vi "Find Songs By Artist.vi"(8 "error in (no error)":errorcluster, 10 "Artist":string, 11 "MusicLibrary in":refnum<class "MusicLibrary.lvclass">) -> (0 "error out":errorcluster, 2 "Songs":refnum<class "Song.lvclass">[](array[class]), 3 "MusicLibrary out":refnum<class "MusicLibrary.lvclass">, 5 "Found?":bool)   [LabVIEW 2015, in "MusicLibrary.lvclass"]
uses:
  MusicLibrary.lvclass
  Song/Song.lvclass
  MusicElementLibrary.lvclass/MusicElementLibrary.ctl
  SongLibrary/SongLibrary.lvclass
  Album/Album.lvclass/Album.ctl
  Song/Song.lvclass/Song.ctl
  MusicElement.lvclass
  MusicElementLibrary.lvclass
  Album/Album.lvclass
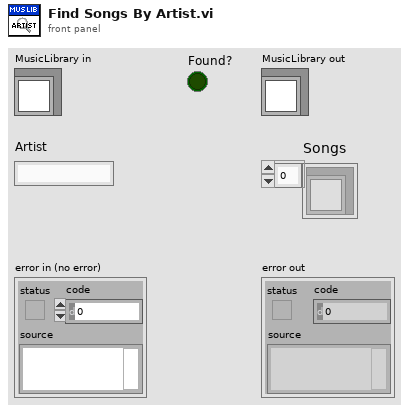
[diagram p1: front panel]
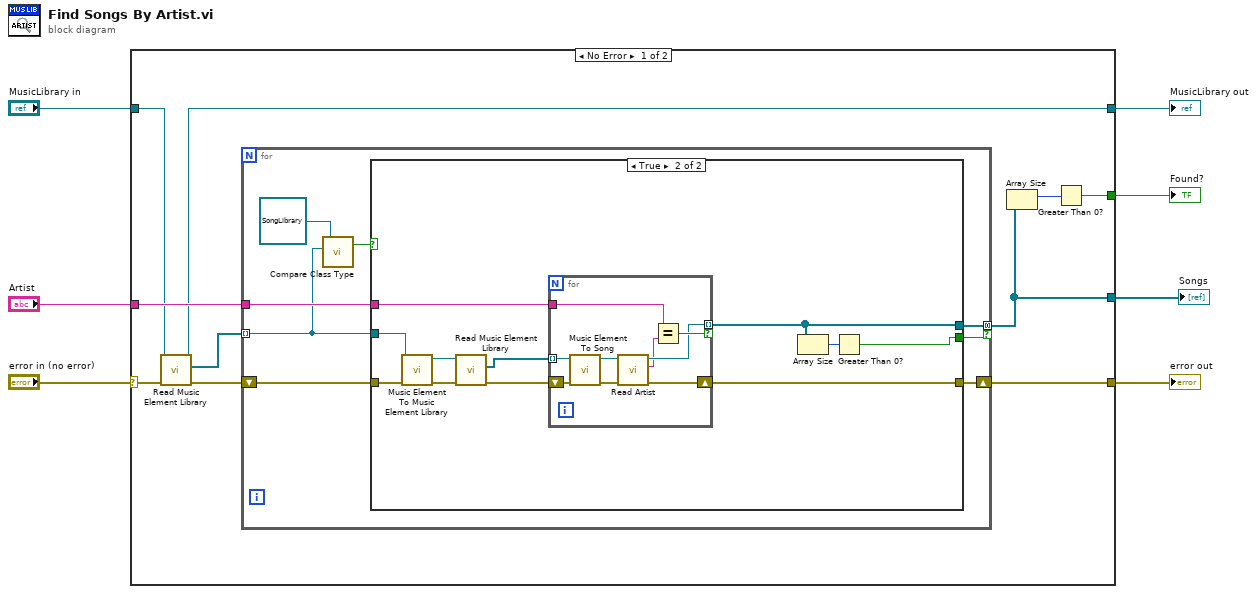
[diagram p0: block diagram]
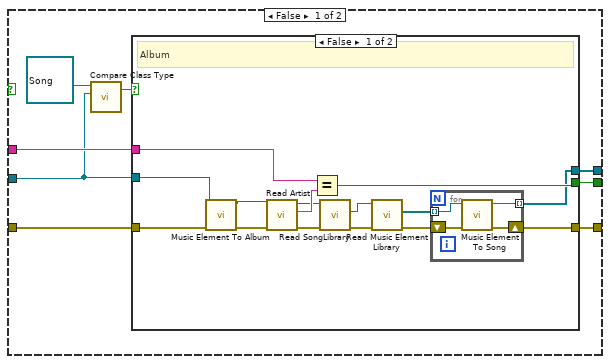
[diagram p2: hidden frame]
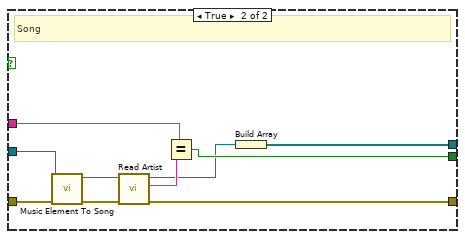
[diagram p3: hidden frame]
diagram:
  n1 = case shown="No Error" "error in (no error)" {
    selector: "error in (no error)" -> [w14 w84]
    tunnel: [w9 w84] -> w6
    tunnel: [w11 w83] -> w4
    tunnel: "MusicLibrary in" -> [w12 w83]
    tunnel: "Artist" -> [w15 _]
    tunnel: [w16 _] -> w2
    tunnel: [w8 _] -> w1
    frame No Error {
      n2 = call "Read Music Element Library.vi"("error in (no error)"=w14, "MusicElementLibrary in"=w12) -> ("error out"=w13:errorcluster, "Music Element Library"=w10:refnum<class "MusicElement.lvclass">[], "MusicElementLibrary out"=w11:refnum<class "MusicLibrary.lvclass">)  [unwired: 7 in]
      n3 = for {
        shift-right: [w25] -> w9
        shift-left: w13 -> [w21]
        tunnel: w15 -> [w24]
        tunnel: w10 -> [w19] mode=indexing
        tunnel: [w23] -> w8 mode=concatenating if=w22
        n4 = call "Compare Class Type.vi"("MusicElement Check"=w19, "MusicElement in"=refnum<class "SongLibrary.lvclass"> refnum ("SongLibrary.lvclass")) -> ("Same Class Type?"=w18:bool)  [unwired: 3 in]
        n5 = case shown="True" w18 {
          tunnel: [w33 w66] -> w25
          tunnel: w24 -> [w32 w67]
          tunnel: [w31 w64] -> w23
          tunnel: [w30 w63] -> w22
          tunnel: w19 -> [w28 w72]
          tunnel: w21 -> [w27 w73]
          frame False {
            n6 = call "Compare Class Type.vi"("MusicElement Check"=w28, "MusicElement in"=refnum<class "Song.lvclass"> refnum ("Song out")) -> ("Same Class Type?"=w26:bool)  [unwired: 3 in]
            n7 = case shown="False" w26 {
              tunnel: [w42 w62] -> w33
              tunnel: w32 -> [w44 w61]
              tunnel: [w35 w58] -> w31
              tunnel: w28 -> [w47 w54]
              tunnel: [w43 w59] -> w30
              tunnel: w27 -> [w34 w56]
              frame False {
                # "Album"
                n8 = call "Music Element To Album.vi"("error in (no error)"=w34, "MusicElement"=w47) -> ("error out"=w48:errorcluster, "Album"=w46:refnum<class "Album.lvclass">)  [unwired: 8 in]
                n9 = call "Read Artist.vi"("error in (no error)"=w48, "Album in"=w46) -> ("error out"=w41:errorcluster, "Artist"=w45:string, "Album out"=w40:refnum<class "Album.lvclass">)  [unwired: 7 in]
                n10 = Equal?(x=w44, y=w45) -> (x = y?=w43:bool)
                n11 = call "Read SongLibrary.vi"("error in (no error)"=w41, "Album in"=w40) -> ("error out"=w39:errorcluster, "SongLibrary.lvclass"=w38:refnum<class "SongLibrary.lvclass">)  [unwired: 7 in, 1 out]
                n12 = call "Read Music Element Library.vi"("error in (no error)"=w39, "MusicElementLibrary in"=w38) -> ("error out"=w36:errorcluster, "Music Element Library"=w37:refnum<class "MusicElement.lvclass">[])  [unwired: 7 in, 1 out]
                n13 = for {
                  shift-right: [w51] -> w42
                  shift-left: w36 -> [w52]
                  tunnel: w37 -> [w50] mode=indexing
                  tunnel: [w49] -> w35 mode=indexing
                  n14 = call "Music Element To Song.vi"("error in (no error)"=w52, "MusicElement"=w50) -> ("error out"=w51:errorcluster, "Song out"=w49:refnum<class "Song.lvclass">)  [unwired: 8 in]
                }
              }
              frame True {
                # "Song"
                n15 = call "Music Element To Song.vi"("error in (no error)"=w56, "MusicElement"=w54) -> ("error out"=w55:errorcluster, "Song out"=w53:refnum<class "Song.lvclass">)  [unwired: 8 in]
                n16 = call "Read Artist.vi"("error in (no error)"=w55, "Song in"=w53) -> ("error out"=w62:errorcluster, "Artist"=w60:string, "Song out"=w57:refnum<class "Song.lvclass">)  [unwired: 7 in]
                n17 = Equal?(x=w61, y=w60) -> (x = y?=w59:bool)
                n18 = Build Array(w57) -> (w58:refnum<class "Song.lvclass">[])
              }
            }
          }
          frame True {
            n19 = call "Music Element To Music Element Library.vi"("error in (no error)"=w73, "MusicElement"=w72) -> ("error out"=w71:errorcluster, "MusicElementLibrary out"=w70:refnum<class "MusicElementLibrary.lvclass">)  [unwired: 8 in]
            n20 = call "Read Music Element Library.vi"("error in (no error)"=w71, "MusicElementLibrary in"=w70) -> ("error out"=w69:errorcluster, "Music Element Library"=w68:refnum<class "MusicElement.lvclass">[])  [unwired: 7 in, 1 out]
            n21 = for {
              tunnel: w68 -> [w80] mode=indexing
              tunnel: w67 -> [w82]
              tunnel: [w75] -> w64 mode=indexing if=w79
              shift-right: [w77] -> w66
              shift-left: w69 -> [w81]
              n22 = call "Music Element To Song.vi"("error in (no error)"=w81, "MusicElement"=w80) -> ("error out"=w78:errorcluster, "Song out"=w76:refnum<class "Song.lvclass">)  [unwired: 8 in]
              n23 = call "Read Artist.vi"("error in (no error)"=w78, "Song in"=w76) -> ("error out"=w77:errorcluster, "Artist"=w74:string, "Song out"=w75:refnum<class "Song.lvclass">)  [unwired: 7 in]
              n24 = Equal?(x=w82, y=w74) -> (x = y?=w79:bool)
            }
            n25 = Array Size(array=w64) -> (size(s)=w65:i32)
            n26 = Greater Than 0?(x=w65) -> (x > 0?=w63:bool)
          }
        }
      }
      n27 = Array Size(array=w8) -> (size(s)=w17:i32)
      n28 = Greater Than 0?(x=w17) -> (x > 0?=w16:bool)
    }
    frame Error {
    }
  }
  "error out" <- w6
  "MusicLibrary out" <- w4
  "Found?" <- w2
  "Songs" <- w1
